vi "WavetoXYData(SGL).vi"(8 "error in (no error)":errorcluster caption="エラー入力（エラーなし）", 10 "StartX":dbl, 11 "WaveForm":waveform(sgl)) -> (0 "error out":errorcluster caption="エラー出力", 3 "XY Cluster":cluster{"X":sgl[], "Y":sgl[]})   [LabVIEW 2015]
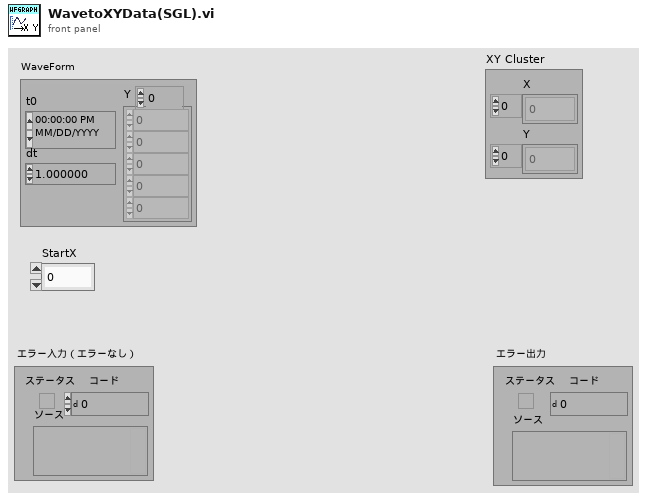
[diagram p1: front panel]
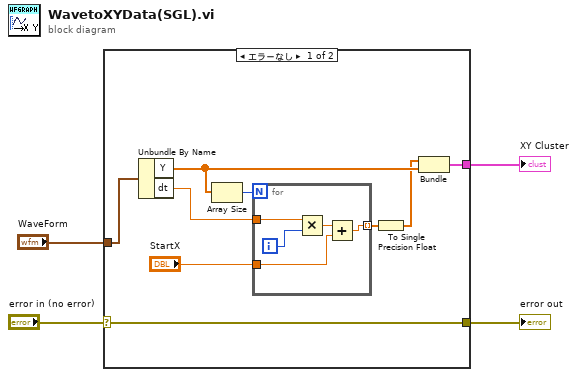
[diagram p0: block diagram]
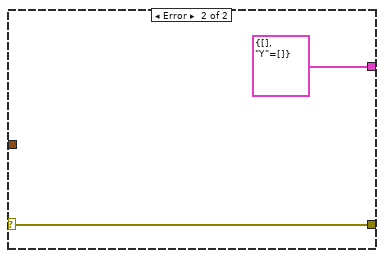
[diagram p2: hidden frame]
diagram:
  n1 = case shown="エラーなし" "error in (no error)" {
    selector: "error in (no error)" -> [w11 w20]
    tunnel: [w11 w20] -> w3
    tunnel: "WaveForm" -> [w13 _]
    tunnel: [w8 cluster{sgl[], "Y":sgl[]} {[], "Y"=[]}] -> w1
    frame No Error {
      n2 = Unbundle By Name(w13) -> ("Y"=w9:sgl[], "dt"=w12:dbl)
      n3 = Array Size(array=w9) -> (size(s)=w10:i32)
      n4 = for {
        N: w10 -> [_]
        tunnel: w12 -> [w18]
        tunnel: [w15] -> w7 mode=indexing
        tunnel: "StartX" -> [w14]
        i -> [w17]
        n5 = Multiply(x=w18, y=w17) -> (x*y=w16:dbl)
        n6 = Add(x=w16, y=w14) -> (x+y=w15:dbl)
      }
      n7 = To Single Precision Float(number=w7) -> (single precision float=w6:sgl[])
      n8 = Bundle(w6, "Y"=w9) -> (w8:cluster{sgl[], "Y":sgl[]})  [unwired: 1 in]
    }
    frame Error {
    }
  }
  "error out" <- w3
  "XY Cluster" <- w1
